vi "setChannel.vi"(8 "error in (no error)":errorcluster, 10 "channel":i32=1, 11 "Tv in":refnum<class "Tv.lvclass">) -> (0 "error out":errorcluster, 3 "Tv out":refnum<class "Tv.lvclass">)   [LabVIEW 2018, in "Tv.lvclass"]
uses:
  Tv.lvclass
  Tv.lvclass/Tv.ctl
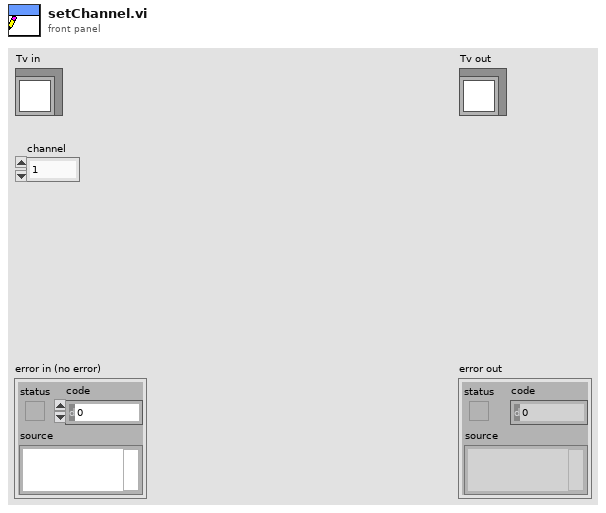
[diagram p1: front panel]
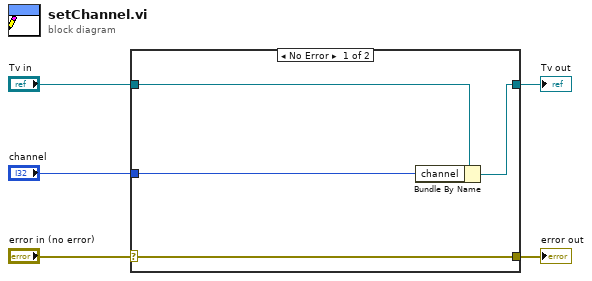
[diagram p0: block diagram]
diagram:
  n1 = case shown="No Error" "error in (no error)" {
    selector: "error in (no error)" -> [w9 w10]
    tunnel: [w9 w10] -> w4
    tunnel: [w7 w11] -> w2
    tunnel: "Tv in" -> [w8 w11]
    tunnel: "channel" -> [w6 _]
    frame No Error {
      n2 = Bundle By Name(cluster=w8, "channel"=w6) -> (w7:refnum<class "Tv.lvclass">)
    }
    frame Error {
    }
  }
  "error out" <- w4
  "Tv out" <- w2
